vi "Send Notification.vi"(8 "error in (no error)":errorcluster, 9 "Timeout":i32, 10 "Notification":variant, 11 "SEQ I64 in":refnum<class "SEQ I64.lvclass">) -> (0 "error out":errorcluster, 1 "Timeout?":bool, 3 "SEQ I64 out":refnum<class "SEQ I64.lvclass">)   [LabVIEW 2022 SP3, in "SEQ I64.lvclass"]
uses:
  SEQ I64.lvclass
  SEQ I64.lvclass/SEQ I64.ctl
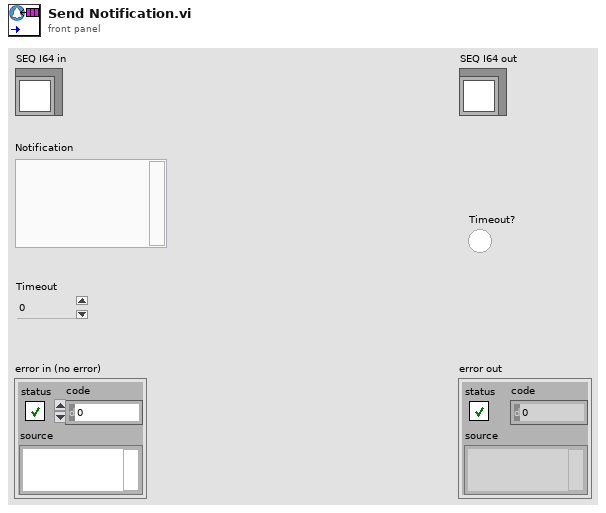
[diagram p1: front panel]
types:
  T1 = typedef "Control 2.ctl" = refnum<queue>
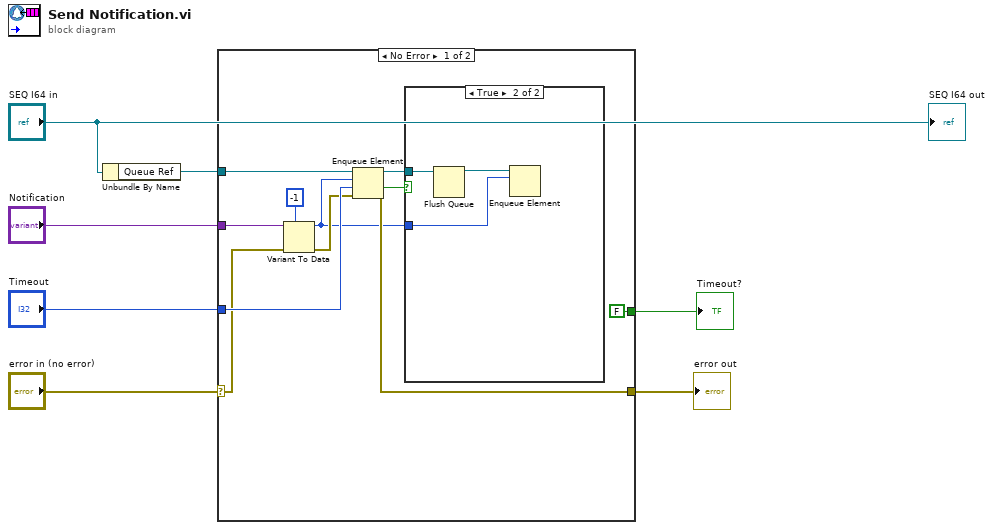
[diagram p0: block diagram]
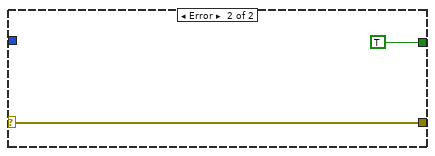
[diagram p3: hidden frame]
diagram:
  n1 = Unbundle By Name("SEQ I64 in") -> ("Queue Ref"=w5:T1)
  n2 = case shown="No Error" "error in (no error)" {
    selector: "error in (no error)" -> [w15 w23]
    tunnel: w5 -> [w18 _]
    tunnel: "Timeout" -> [w17 _]
    tunnel: "Notification" -> [w16 _]
    tunnel: [w9 w23] -> w2
    tunnel: [FALSE ("timed out?") TRUE ("timed out?")] -> w1
    frame No Error {
      n3 = Variant To Data(error in=w15, type=i64 -1 ("Timeout"), Variant=w16) -> (data=w8:i64, error out=w14:errorcluster)
      n4 = Enqueue Element(queue=w18, element=w8, timeout in ms (-1)=w17, error in (no error)=w14) -> (queue out=w11:T1, timed out?=w12:bool, error out=w9:errorcluster)
      n5 = case shown="True" w12 {
        tunnel: w11 -> [_ w21]
        tunnel: w8 -> [_ w19]
        frame False {
        }
        frame True {
          n6 = Flush Queue(queue=w21) -> (queue out=w20:T1)  [unwired: 1 in, 2 out]
          n7 = Enqueue Element(queue=w20, element=w19) -> ()  [unwired: 2 in, 3 out]
        }
      }
    }
    frame Error {
    }
  }
  "error out" <- w2
  "Timeout?" <- w1
  "SEQ I64 out" <- "SEQ I64 in"
